vi "Untitled 2 (SubVI) 1.vi"() -> (3 "Cluster":cluster{dbl, dbl, dbl, dbl, dbl, string})   [LabVIEW 2014]
doc: "Put default value of our pecer"
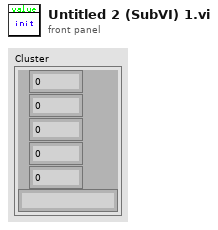
[diagram p1: front panel]
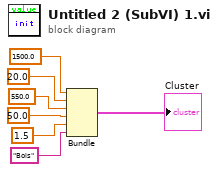
[diagram p0: block diagram]
diagram:
  n1 = Bundle(1500.0, 20.0, 550.0, 50.0, 1.5, "Bois") -> (→"Cluster":cluster{dbl, dbl, dbl, dbl, dbl, string})  [unwired: 1 in]
